vi "Bayer.vi"(9 "Height":i32, 10 "Width":i32, 11 "Array":u8[](array[numeric])) -> (3 "new picture":picture)   [LabVIEW 2015]
uses:
  <vilib>/picture/picture.llb/Draw True-Color Pixmap.vi
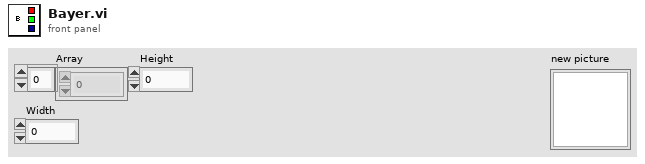
[diagram p1: front panel]
types:
  T1 = cluster{"LT":u16, "T":u16, "RT":u16, "L":u16, "X":u16, "R":u16, "LB":u16, "B":u16, "RB":u16}
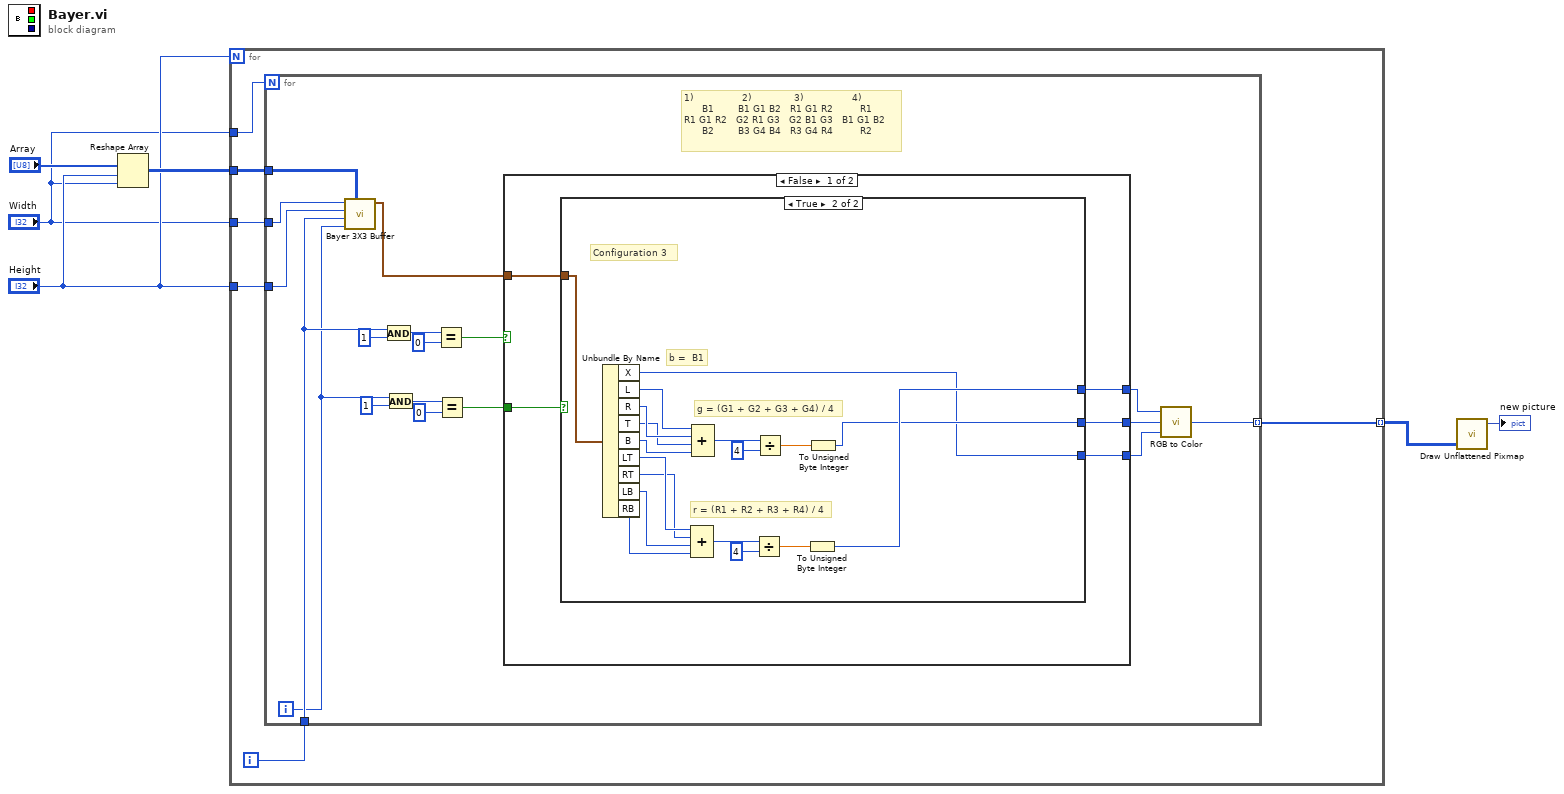
[diagram p0: block diagram]
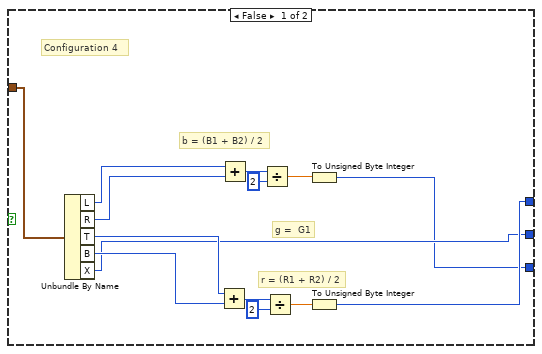
[diagram p2: hidden frame]
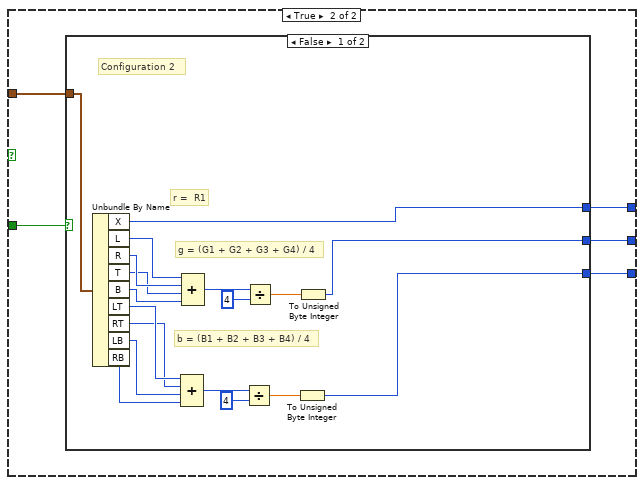
[diagram p3: hidden frame]
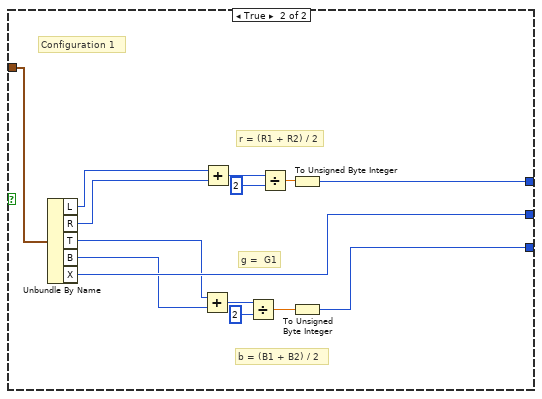
[diagram p4: hidden frame]
diagram:
  n1 = Reshape Array("Array", "Height", "Width") -> (w5:u8[][])
  n2 = for {
    N: "Height" -> [_]
    tunnel: w5 -> [w11]
    tunnel: "Width" -> [w12]
    tunnel: "Width" -> [w10]
    tunnel: "Height" -> [w9]
    tunnel: [w7] -> w4 mode=indexing
    i -> [w8]
    n3 = for {
      N: w12 -> [_]
      tunnel: w11 -> [w30]
      tunnel: w10 -> [w29]
      tunnel: w9 -> [w28]
      tunnel: w8 -> [w27]
      tunnel: [w13] -> w7 mode=indexing
      i -> [w25]
      # "1)                2)              3)                4)\n      B1        B1 G1 B2   R1 G1 R2         R1\nR1 G1 R2   G2 R1 G3   G2 B1 G3   B1 G1 B2 \n      B2        B3 G4 B4   R3 G4 R4         R2"
      n4 = call "Bayer 3X3 Buffer.vi"("Bayer Array"=w30, "Col Inde"=w25, "Row Index"=w27, "Height"=w28, "Width"=w29) -> ("3X3 Buffer"=w17:T1)  [unwired: 6 in]
      n5 = And(x=w27, y=1) -> (x .and. y?=w23:i32)
      n6 = And(x=w25, y=1) -> (x .and. y?=w21:i32)
      n7 = Equal?(x=w23, y=0) -> (x = y?=w19:bool)
      n8 = Equal?(x=w21, y=0) -> (x = y?=w18:bool)
      n9 = case shown="False" w19 {
        tunnel: w18 -> [w34 w72]
        tunnel: w17 -> [w35 w71]
        tunnel: [w33 w70] -> w16
        tunnel: [w32 w69] -> w15
        tunnel: [w31 w68] -> w14
        frame False {
          n10 = case shown="True" w34 {
            tunnel: w35 -> [w36 w53]
            tunnel: [w39 w52] -> w33
            tunnel: [w38 w51] -> w32
            tunnel: [w37 w50] -> w31
            frame False {
              # "g =  G1"
              # "b = (B1 + B2) / 2"
              # "r = (R1 + R2) / 2"
              # "Configuration 4"
              n11 = Unbundle By Name(w36) -> ("L"=w49:u16, "R"=w48:u16, "T"=w44:u16, "B"=w43:u16, "X"=w38:u16)
              n12 = Add(x=w44, y=w43) -> (x+y=w40:u16)
              n13 = Add(x=w49, y=w48) -> (x+y=w47:u16)
              n14 = Divide(x=w47, y=u16 2) -> (x/y=w45:dbl)
              n15 = Divide(x=w40, y=u16 2) -> (x/y=w41:dbl)
              n16 = To Unsigned Byte Integer(number=w45) -> (unsigned 8bit integer=w37:u8)
              n17 = To Unsigned Byte Integer(number=w41) -> (unsigned 8bit integer=w39:u8)
            }
            frame True {
              # "r = (R1 + R2 + R3 + R4) / 4"
              # "g = (G1 + G2 + G3 + G4) / 4"
              # "b =  B1"
              # "Configuration 3"
              n18 = Unbundle By Name(w53) -> ("X"=w50:u16, "L"=w67:u16, "R"=w66:u16, "T"=w65:u16, "B"=w64:u16, "LT"=w57:u16, "RT"=w56:u16, "LB"=w55:u16, "RB"=w54:u16)
              n19 = Compound Arithmetic op=ADD(w57, w56, w55, w54) -> (w60:u16)
              n20 = Compound Arithmetic op=ADD(w67, w66, w65, w64) -> (w63:u16)
              n21 = Divide(x=w60, y=u16 4) -> (x/y=w58:dbl)
              n22 = Divide(x=w63, y=u16 4) -> (x/y=w61:dbl)
              n23 = To Unsigned Byte Integer(number=w58) -> (unsigned 8bit integer=w52:u8)
              n24 = To Unsigned Byte Integer(number=w61) -> (unsigned 8bit integer=w51:u8)
            }
          }
        }
        frame True {
          n25 = case shown="False" w72 {
            tunnel: w71 -> [w90 w104]
            tunnel: [w83 w98] -> w70
            tunnel: [w81 w97] -> w69
            tunnel: [w73 w91] -> w68
            frame False {
              # "b = (B1 + B2 + B3 + B4) / 4"
              # "g = (G1 + G2 + G3 + G4) / 4"
              # "r =  R1"
              # "Configuration 2"
              n26 = Unbundle By Name(w90) -> ("X"=w83:u16, "L"=w89:u16, "R"=w88:u16, "T"=w87:u16, "B"=w86:u16, "LT"=w77:u16, "RT"=w76:u16, "LB"=w75:u16, "RB"=w74:u16)
              n27 = Compound Arithmetic op=ADD(w77, w76, w75, w74) -> (w80:u16)
              n28 = Compound Arithmetic op=ADD(w89, w88, w87, w86) -> (w85:u16)
              n29 = Divide(x=w80, y=u16 4) -> (x/y=w78:dbl)
              n30 = Divide(x=w85, y=u16 4) -> (x/y=w82:dbl)
              n31 = To Unsigned Byte Integer(number=w78) -> (unsigned 8bit integer=w73:u8)
              n32 = To Unsigned Byte Integer(number=w82) -> (unsigned 8bit integer=w81:u8)
            }
            frame True {
              # "b = (B1 + B2) / 2"
              # "g =  G1"
              # "r = (R1 + R2) / 2"
              # "Configuration 1"
              n33 = Unbundle By Name(w104) -> ("L"=w103:u16, "R"=w102:u16, "T"=w96:u16, "B"=w95:u16, "X"=w97:u16)
              n34 = Add(x=w96, y=w95) -> (x+y=w94:u16)
              n35 = Add(x=w103, y=w102) -> (x+y=w101:u16)
              n36 = Divide(x=w94, y=u16 2) -> (x/y=w92:dbl)
              n37 = Divide(x=w101, y=u16 2) -> (x/y=w99:dbl)
              n38 = To Unsigned Byte Integer(number=w99) -> (unsigned 8bit integer=w98:u8)
              n39 = To Unsigned Byte Integer(number=w92) -> (unsigned 8bit integer=w91:u8)
            }
          }
        }
      }
      n40 = call <vilib>:"RGB to Color.vi"("B"=w14, "G"=w15, "R"=w16) -> ("Color"=w13:u32)
    }
  }
  n41 = call-poly <vilib>:"Draw Unflattened Pixmap.vi"("data (RGB format)"=w4) -> ("new picture"=→"new picture":picture)  [unwired: 8 in]
